vi "Create Progect.vi"(1 "Source DIR":path, 2 "element":string, 3 "selected path":path) -> (0 "Boolean":bool)   [LabVIEW 2010]
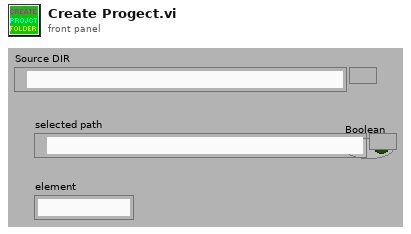
[diagram p1: front panel]
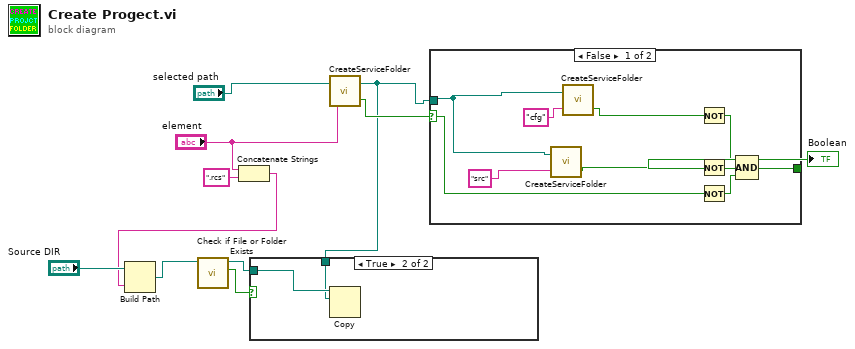
[diagram p0: block diagram]
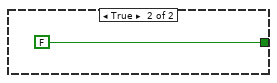
[diagram p3: hidden frame]
diagram:
  n1 = Concatenate Strings("element", ".rcs" ("string")) -> (w5:string)
  n2 = Build Path(base path="Source DIR", name or relative path=w5) -> (appended path=w4:path)
  n3 = call <vilib>:"Check if File or Folder Exists.vi"("path"=w4) -> ("file or folder exists?"=w3:bool, "dup path"=w1:path)  [unwired: 8 in, 1 out]
  n4 = call "CreateServiceFolder.vi"("element"="element", "selected path"="selected path") -> ("cancelled"=w10:bool, "created path"=w2:path)
  n5 = case shown="True" w3 {
    tunnel: w2 -> [_ w12]
    tunnel: w1 -> [_ w13]
    frame False {
    }
    frame True {
      n6 = Copy(10:w12, 11:w13) -> ()  [unwired: 3 in, 3 out]
    }
  }
  n7 = case shown="False" w10 {
    selector: w10 -> [w20 _]
    tunnel: w2 -> [w16 _]
    tunnel: [w19 FALSE] -> w11
    frame False {
      n8 = call "CreateServiceFolder.vi"("element"="src" ("prompt (Create Folder)"), "selected path"=w16) -> ("cancelled"=w14:bool)  [unwired: 1 out]
      n9 = call "CreateServiceFolder.vi"("element"="cfg" ("prompt (Create Folder)"), "selected path"=w16) -> ("cancelled"=w17:bool)  [unwired: 1 out]
      n10 = Not(x=w17) -> (.not. x?=w23:bool)
      n11 = Not(x=w14) -> (.not. x?=w22:bool)
      n12 = Not(x=w20) -> (.not. x?=w21:bool)
      n13 = Compound Arithmetic op=AND(w23, w22, w21) -> (w19:bool)
    }
    frame True {
    }
  }
  "Boolean" <- w11
